vi "Split Array index for Parallel Code.vi"(8 "Array Size":i32) -> (0 "Length3":i32, 1 "Index3":i32, 2 "Length2":i32, 3 "Index2":i32, 4 "Index4":i32, 5 "Length1":i32, 6 "Length4":i32, 7 "Index1":i32)   [LabVIEW 2022 SP3]
panel:
  in  "No Of Loops":i32=4
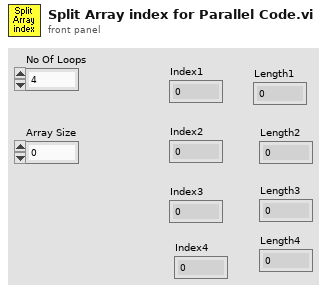
[diagram p1: front panel]
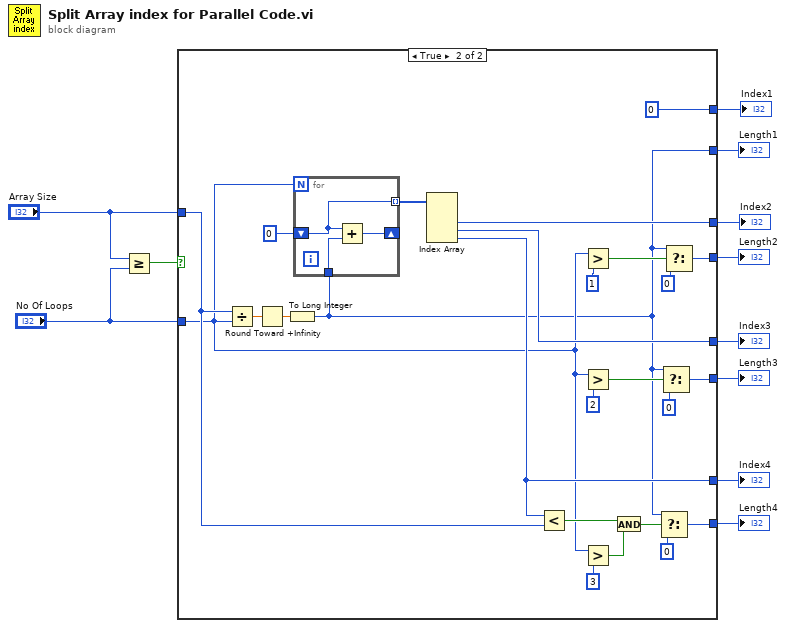
[diagram p0: block diagram]
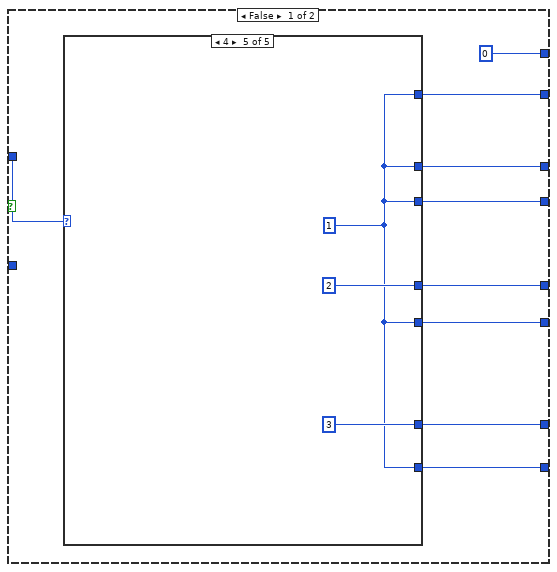
[diagram p2: hidden frame]
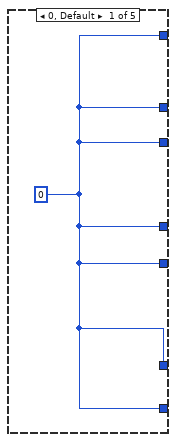
[diagram p3: hidden frame]
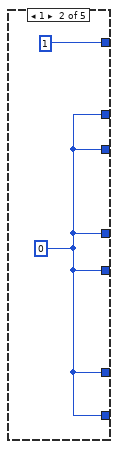
[diagram p4: hidden frame]
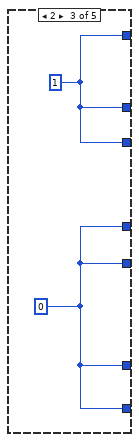
[diagram p5: hidden frame]
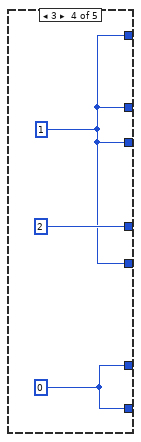
[diagram p6: hidden frame]
diagram:
  n1 = Greater Or Equal?(x="Array Size", y="No Of Loops") -> (x >= y?=w6:bool)
  n2 = case shown="True" w6 {
    tunnel: [w18 w56] -> w11
    tunnel: [w14 w40] -> w10
    tunnel: [w16 w50] -> w9
    tunnel: "Array Size" -> [w20 w51]
    tunnel: "No Of Loops" -> [_ w35]
    tunnel: [w17 w48] -> w5
    tunnel: [w15 w39] -> w4
    tunnel: [w13 w41] -> w3
    tunnel: [w19 w32] -> w2
    tunnel: [0 0] -> w1
    frame False {
      n3 = case shown="4" w20 {
        tunnel: [w21 1 w24 w26 w29] -> w19
        tunnel: [w21 w22 w24 w26 w29] -> w18
        tunnel: [w21 w22 w25 w28 w29] -> w17
        tunnel: [w21 w22 w25 w28 3] -> w16
        tunnel: [w21 w22 w25 w26 w29] -> w15
        tunnel: [w21 w22 w25 2 2] -> w14
        tunnel: [w21 w22 w24 w26 w29] -> w13
        frame 0, Default {
          w21 = 0
        }
        frame 1 {
          w22 = 0
        }
        frame 2 {
          w25 = 0
          w24 = 1
        }
        frame 3 {
          w28 = 0
          w26 = 1
        }
        frame 4 {
          w29 = 1
        }
      }
    }
    frame True {
      n4 = Divide(x=w51, y=w35) -> (x/y=w53:dbl)
      n5 = Round Toward +Infinity(x=w53) -> (ceil(x): smallest int >= x=w52:dbl)
      n6 = To Long Integer(number=w52) -> (32bit integer=w32:i32)
      n7 = for {
        N: w35 -> [_]
        shift-right: [w58] -> _
        shift-left: 0 -> [w57]
        tunnel: w32 -> [w59]
        tunnel: [w57] -> w55 mode=indexing
        n8 = Add(x=w57, y=w59) -> (x+y=w58:i32)
      }
      n9 = Index Array(array=w55) -> (element #2=w56:i32, element #3=w40:i32, element #4=w50:i32)  [unwired: 4 in, 1 out]
      n10 = Less?(x=w50, y=w51) -> (x < y?=w38:bool)
      n11 = Greater?(x=w35, y=1) -> (0:w46:bool)
      n12 = Greater?(x=w35, y=2) -> (0:w43:bool)
      n13 = Greater?(x=w35, y=3) -> (0:w34:bool)
      n14 = And(x=w38, y=w34) -> (x .and. y?=w37:bool)
      n15 = Select(t=w32, s=w37, f=0) -> (s? t:f=w48:i32)
      n16 = Select(t=w32, s=w43, f=0) -> (s? t:f=w39:i32)
      n17 = Select(t=w32, s=w46, f=0) -> (s? t:f=w41:i32)
    }
  }
  "Length1" <- w2
  "Index2" <- w11
  "Index3" <- w10
  "Index4" <- w9
  "Index1" <- w1
  "Length2" <- w3
  "Length3" <- w4
  "Length4" <- w5
